vi "MonitorLoop.vi"(0 "C space":refnum<vi>, 5 "D space":refnum<vi>) -> ()   [LabVIEW 2020, in "DiskSpaceMonitor.xctl"]
uses:
  DiskSpaceMonitor.xctl
  <vilib>/Platform/TimedLoop/XDataNode/timing_clust.ctl
  <vilib>/Platform/TimedLoop/XDataNode/nitl_modes.ctl
  <vilib>/Platform/TimedLoop/XDataNode/wakeup.ctl
  <vilib>/platform/TimedLoop/XDataNode/XDataNode.xnode
  <vilib>/Platform/TimedLoop/XDataNode/XDNodeRunTimeDep.lvlib
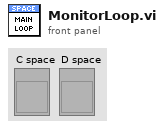
[diagram p1: front panel]
types:
  T1 = typedef "XDNodeRunTimeDep.lvlib/timing_clust.ctl" = cluster{"Expected End [f-1]":u64, "Actual End [f-1]":u64, "Finished Late? [f-1]":bool, "Expected End [i-1]":u64, "Actual End [i-1]":u64, "Finished Late? [i-1]":bool, "Expected Start [i]":u64, "Actual Start [i]":u64, "Expected Start [f]":u64, "Actual Start [f]":u64, "Source Name":string, "Structure Name":string, "Period":i64, "Deadline":i64, "Offset":i64, "Start":i64, "Priority":i32, "Timeout":i32, "Mode":T2, "Wakeup Reason":T3, "Error":errorcluster, "Source Type":string, "Secondary Source Type":string, "Global End Time":u64, "Global Start Time":u64, "Frame Duration":u64, "Iteration Duration":u64, "Assigned CPU":i32, "I/O Scan Engine Mode":u32}
  T2 = typedef "XDNodeRunTimeDep.lvlib/nitl_modes.ctl" = enum32{"No Change", "Process missed periods, maintain original phase", "Discard missed periods, maintain original phase", "Process missed periods, ignore original phase", "Discard missed periods, ignore original phase"}
  T3 = typedef "XDNodeRunTimeDep.lvlib/wakeup.ctl" = enum32{"Normal", "Aborted", "Asynchronous wakeup", "Timing source error", "Timed loop error", "Timeout"}
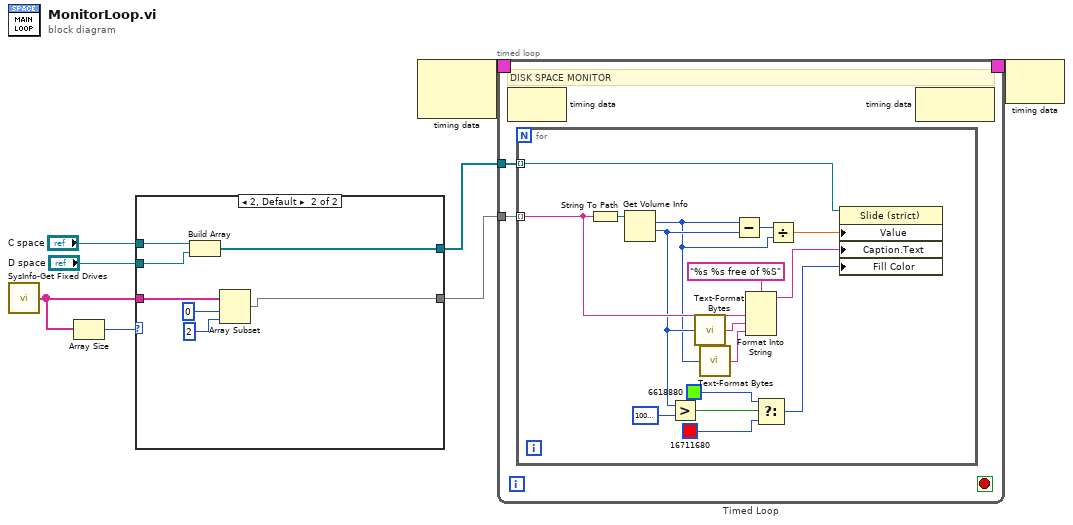
[diagram p0: block diagram]
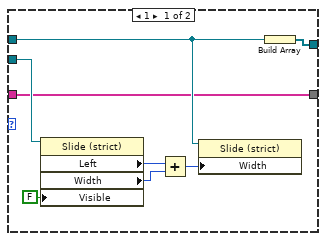
[diagram p2: hidden frame]
diagram:
  n1 = call "SysInfo-Get Fixed Drives.vi"() -> ("Fixed drives"=w1:string[])  [unwired: 14 in, 1 out]
  n2 = Array Size(array=w1) -> (size(s)=w2:i32)
  n3 = case shown="2, Default" w2 {
    tunnel: "C space" -> [w12 w23]
    tunnel: "D space" -> [w15 w22]
    tunnel: [w16 w21] -> w4
    tunnel: [w9 w17] -> w3
    tunnel: w1 -> [w9 w20]
    frame 1 {
      n4 = property class="Slide (strict)"(reference=w15, "Visible"=FALSE) -> ("Left"=w13:i32, "Width"=w14:u32)  [unwired: 1 in, 2 out]
      n5 = Add(x=w13, y=w14) -> (x+y=w11:u32)
      n6 = property class="Slide (strict)"(reference=w12, "Width"=w11) -> ()  [unwired: 1 in, 2 out]
      n7 = Build Array(w12) -> (w16:refnum<vi>[])
    }
    frame 2, Default {
      n8 = Build Array(w23, w22) -> (w21:refnum<vi>[])
      n9 = Array Subset(array=w20, index=0, length=2) -> (w17:string[])
    }
  }
  n10 = node-c288() -> (w8:T1)  [unwired: 2 in]
  n11 = timed-loop "Timed Loop" {
    timing: w8 -> [_]
    timing-out: [_] -> w7
    tunnel: w3 -> [w25]
    tunnel: w4 -> [w24]
    stop <- _ stop-if-true
    # "DISK SPACE MONITOR"
    n12 = node-c288() -> ()  [unwired: 1 in, 1 out]
    n13 = for {
      tunnel: w25 -> [w40] mode=indexing
      tunnel: w24 -> [w41] mode=indexing
      n14 = String To Path(string=w40) -> (path=w38:path)
      n15 = Get Volume Info(11:w38) -> (1:w29:i64, 2:w27:i64)  [unwired: 1 in, 4 out]
      n16 = Greater?(x=w29, y=i64 10000000000) -> (0:w35:bool)
      n17 = call "Text-Format Bytes.vi"("Bytes"=w29) -> ("resulting string"=w28:string)  [unwired: 14 in]
      n18 = call "Text-Format Bytes.vi"("Bytes"=w27) -> ("resulting string"=w26:string)  [unwired: 14 in]
      n19 = Subtract(x=w27, y=w29) -> (x-y=w39:i64)
      n20 = Format Into String(format string="%s %s free of %S", w40, w28, w26) -> (resulting string=w31:string)  [unwired: 2 in, 1 out]
      n21 = Select(t=u32 6618880, s=w35, f=u32 16711680) -> (s? t:f=w30:u32)
      n22 = Divide(x=w39, y=w27) -> (x/y=w32:dbl)
      n23 = property class="Slide (strict)"(reference=w41, "Value"=w32, "Caption.Text"=w31, "Fill Color"=w30) -> ()  [unwired: 1 in, 2 out]
    }
    n24 = node-c288() -> ()  [unwired: 1 in, 1 out]
  }
  n25 = node-c288(w7) -> ()  [unwired: 1 out]
